vi "Initialize with Switch Parameters Core.vi"(8 "error in (no error)":errorcluster, 10 "Switch Parameters in":refnum<class "Abstract Switch Init Parameters.lvclass">, 11 "SLSC Switch Consumer in":refnum<class "NI-SWITCH Consumer.lvclass">=refnum) -> (0 "error out":errorcluster, 3 "SLSC Switch Consumer out":refnum<class "NI-SWITCH Consumer.lvclass">)   [LabVIEW 2017, in "NI-SWITCH Messaging.lvlib" / "NI-SWITCH Consumer.lvclass"]
uses:
  NI-SWITCH Consumer.lvclass
  Includes/CDMessaging.lvlibp/Switch/Abstract Switch Init Parameters/Abstract Switch Init Parameters.lvclass
  NI-SWITCH Init Parameters/NI-SWITCH Init Parameters.lvclass
  C:/Dev/GitHub/niveristand-slsc-switch-message-library/Includes/CDMessaging.lvlibp/Switch/Abstract Switch Init Parameters/Abstract Switch Init Parameters.lvclass
  NI-SWITCH Consumer.lvclass/NI-SWITCH Consumer.ctl
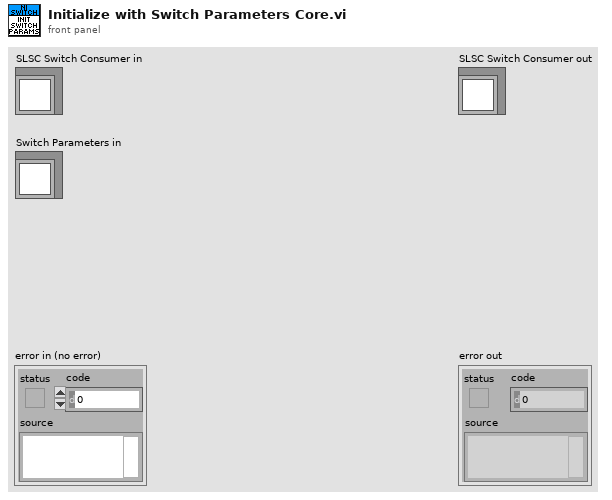
[diagram p1: front panel]
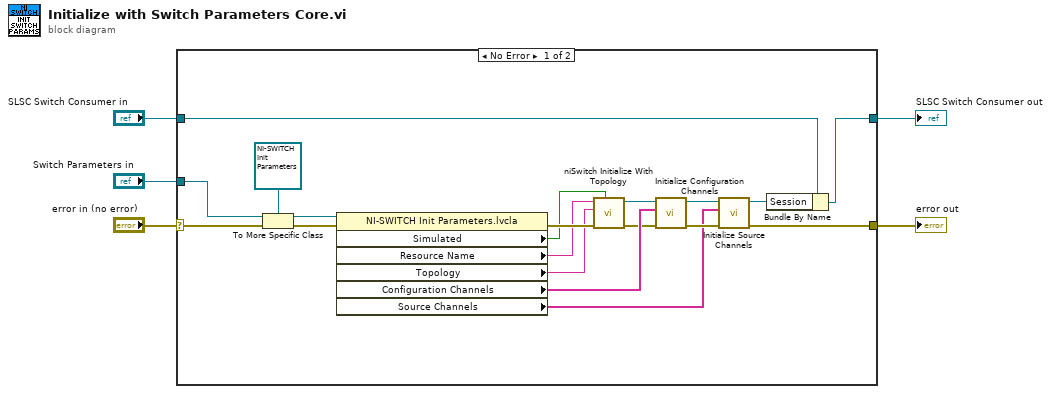
[diagram p0: block diagram]
diagram:
  n1 = case shown="No Error" "error in (no error)" {
    selector: "error in (no error)" -> [w18 w26]
    tunnel: [w13 w26] -> w4
    tunnel: [w23 w25] -> w1
    tunnel: "SLSC Switch Consumer in" -> [w24 w25]
    tunnel: "Switch Parameters in" -> [w21 _]
    frame No Error {
      n2 = To More Specific Class(target class=refnum<class "NI-SWITCH Init Parameters.lvclass"> refnum ("SLSC Switch Messaging.lvlib:SLSC Switch Init Parameters.lvclass"), reference=w21, error in=w18) -> (specific class reference=w19:refnum<class "NI-SWITCH Init Parameters.lvclass">, error out=w17:errorcluster)
      n3 = property class="NI-SWITCH Init Parameters.lvcla"(reference=w19, error in=w17) -> (error out=w22:errorcluster, "Simulated"=w7:bool, "Resource Name"=w6:string, "Topology"=w8:string, "Configuration Channels"=w12:string[], "Source Channels"=w11:string[])  [unwired: 1 out]
      n4 = call <instrlib>:"niSwitch Initialize With Topology.vi"("simulate (boolean value)"=w7, "error in (no error)"=w22, "topology name"=w8, "resource name"=w6) -> ("error out"=w10:errorcluster, "instrument handle out"=w9:refnum<k15>)  [unwired: 6 in]
      n5 = call "Initialize Configuration Channels.vi"("error in (no error)"=w10, "Configuration Channels"=w12, "Session in"=w9) -> ("error out"=w14:errorcluster, "Session out"=w16:refnum<k15>)  [unwired: 7 in]
      n6 = call "Initialize Source Channels.vi"("error in (no error)"=w14, "Source Channels"=w11, "Session in"=w16) -> ("error out"=w13:errorcluster, "Session out"=w15:refnum<k15>)  [unwired: 7 in]
      n7 = Bundle By Name(cluster=w24, "Session"=w15) -> (w23:refnum<class "NI-SWITCH Consumer.lvclass">)
    }
    frame Error {
    }
  }
  "error out" <- w4
  "SLSC Switch Consumer out" <- w1
